vi "niRFSTS DCPower Close.vi"(11 "Semiconductor Module Context":T1) -> (0 "error out":errorcluster)   [LabVIEW 2014]
uses:
  <vilib>/NI_TestStand_SemiconductorModule/NI_TestStand_Semiconductor_Module.lvlibp/PinMap/General/SemiconductorModuleContext.ctl
  <vilib>/NI_TestStand_SemiconductorModule/NI_TestStand_Semiconductor_Module.lvlibp
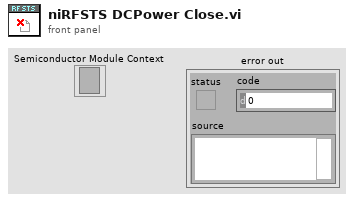
[diagram p1: front panel]
types:
  T1 = typedef "NI_TestStand_Semiconductor_Module.lvlibp/SemiconductorModuleContext.ctl" = refnum<k7>
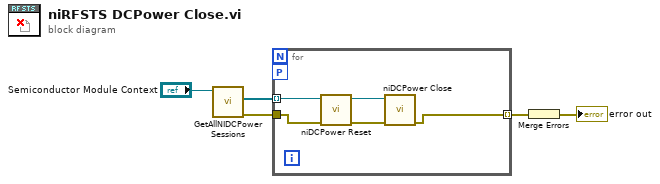
[diagram p0: block diagram]
diagram:
  n1 = call <vilib>:"GetAllNIDCPowerSessions.vi"("Semiconductor Module Context"="Semiconductor Module Context") -> ("error out"=w5:errorcluster, "Instrument Sessions"=w4:refnum<k15>[])  [unwired: 8 in, 1 out]
  n2 = for {
    tunnel: w4 -> [w9] mode=indexing
    workers-P: _ -> [_]
    tunnel: w5 -> [w8]
    tunnel: [w6] -> w1 mode=indexing
    n3 = call <instrlib>:"niDCPower Reset.vi"("error in (no error)"=w8, "instrument handle"=w9) -> ("error out"=w7:errorcluster, "instrument handle out"=w10:refnum<k15>)  [unwired: 8 in]
    n4 = call <instrlib>:"niDCPower Close.vi"("error in (no error)"=w7, "instrument handle"=w10) -> ("error out"=w6:errorcluster)  [unwired: 9 in]
  }
  n5 = Merge Errors(w1) -> (→"error out":errorcluster)
